vi "Get DBL Notifier Ref.vi"(8 "error in (no error)":errorcluster, 9 "element data type":dbl format="%#_13g", 10 "Tag Name":string, 11 "Current Value Table in":refnum<class "Current Value Table.lvclass">) -> (0 "error out":errorcluster, 2 "notifier out":refnum<notifier>, 3 "Current Value Table out":refnum<class "Current Value Table.lvclass">)   [LabVIEW 2024, in "Current Value Table.lvlib" / "Current Value Table.lvclass"]
uses:
  Current Value Table.lvclass
  CVT_DBL/CVT_DBL.lvclass
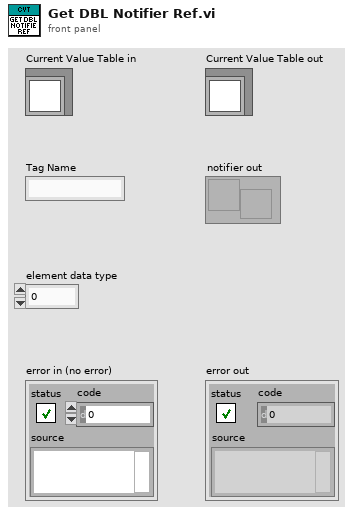
[diagram p1: front panel]
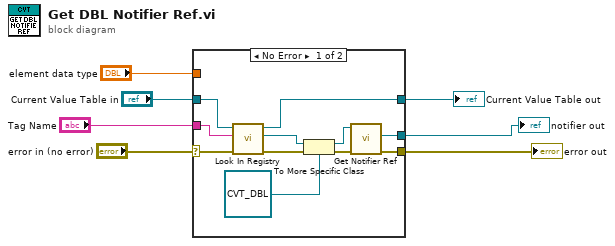
[diagram p0: block diagram]
diagram:
  n1 = case shown="No Error" "error in (no error)" {
    selector: "error in (no error)" -> [w14 w20]
    tunnel: [w10 w20] -> w6
    tunnel: [w8 w19] -> w4
    tunnel: "Current Value Table in" -> [w18 w19]
    tunnel: "Tag Name" -> [w17 _]
    tunnel: [w9 _] -> w2
    tunnel: "element data type" -> [_ _]
    frame No Error {
      n2 = call-dynamic "Look In Registry.vi"("error in (no error)"=w14, "Tag Name"=w17, "Current Value Table in"=w18) -> ("error out"=w15:errorcluster, "CVT_Item out"=w16:refnum<class "iCVT_Item.lvclass">, "Current Value Table out"=w8:refnum<class "Current Value Table.lvclass">)  [unwired: 5 in, 1 out]
      n3 = To More Specific Class(target class=refnum<class "CVT_DBL.lvclass"> refnum ("Current Value Table.lvlib:CVT_DBL.lvclass"), reference=w16, error in=w15) -> (specific class reference=w12:refnum<class "CVT_DBL.lvclass">, error out=w11:errorcluster)
      n4 = call-dynamic "Get Notifier Ref.vi"("error in (no error)"=w11, "CVT_DBL in"=w12) -> ("error out"=w10:errorcluster, "notifier out"=w9:refnum<notifier>)  [unwired: 7 in, 1 out]
    }
    frame Error {
    }
  }
  "error out" <- w6
  "Current Value Table out" <- w4
  "notifier out" <- w2
